vi "Det_Lock_Unlock.vi"(8 "entrée d'erreur (pas d'erreur)":errorcluster, 10 "Control-Client old entrée":refnum<class "Control-Client.lvclass">, 11 "Control-Client new entrée":refnum<class "Control-Client.lvclass">) -> (0 "sortie d'erreur":errorcluster, 2 "Control-Client old out":refnum<class "Control-Client.lvclass">, 3 "Control-Client new out":refnum<class "Control-Client.lvclass">)   [LabVIEW 2019, in "Control-Client.lvclass"]
uses:
  Control-Client.lvclass
  Control-Client.lvclass/Control-Client.ctl
  controls/Gauge_pump/Gauge_pump.xctl
  dependecies/XControls/CellsDL/ControlDL.xctl
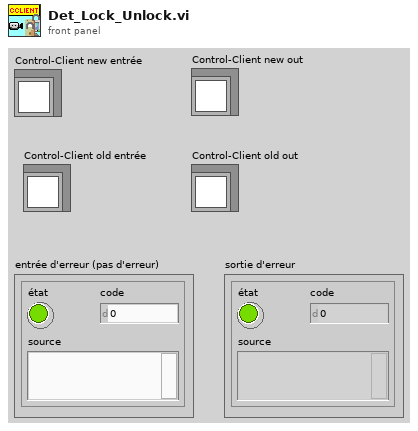
[diagram p1: front panel]
types:
  T1 = enum8{"Enabled", "Disabled", "Disabled and Grayed Out"}
  T2 = typedef "Control-Client.lvclass/Controls-with-permissions_CLIENT.ctl" = cluster{"Server ON/OFF":refnum<vi>, "Detector connect":refnum<vi>, "DL connect":refnum<vi>, "DAQmx connect":refnum<vi>, "All connect":refnum<vi>, "Start measurement":refnum<vi>, "Move Crystal":refnum<vi>, "Relay key heater":refnum<vi>, "Laser Shutter":refnum<vi>, "Accelerator Shutter":refnum<vi>, "Power":refnum<vi>, "Unlock":refnum<vi>, "RT":refnum<vi>, "Faraday Cup":refnum<vi>, "Osc connect":refnum<vi>, "ELYSE pulses":refnum<vi>, "Cells":refnum<vi>, "Pump":refnum<vi>, "# par point":refnum<vi>, "Alarm":refnum<vi>, "oscilloscopeRead":refnum<vi>, "WCM_state":refnum<vi>, "ControlDL":refnum<vi>}
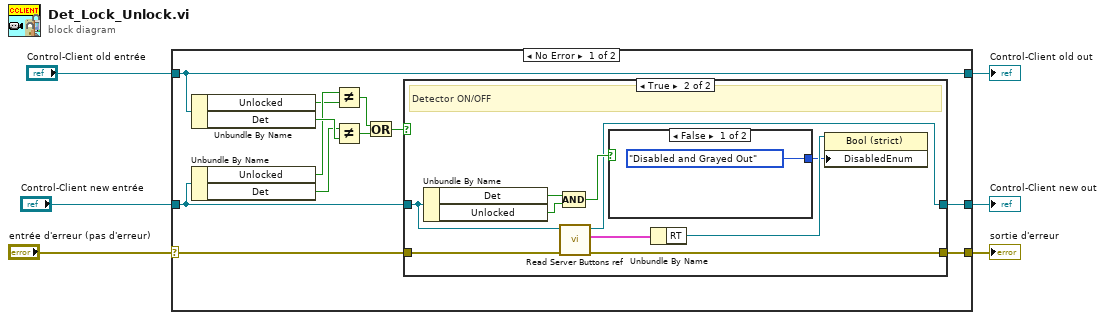
[diagram p0: block diagram]
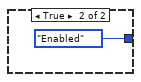
[diagram p3: hidden frame]
diagram:
  n1 = case shown="No Error" "entrée d'erreur (pas d'erreur)" {
    selector: "entrée d'erreur (pas d'erreur)" -> [w8 w33]
    tunnel: [w18 w33] -> w6
    tunnel: "Control-Client new entrée" -> [w17 w35]
    tunnel: "Control-Client old entrée" -> [w7 w34]
    tunnel: [w9 w35] -> w3
    tunnel: [w7 w34] -> w1
    frame No Error {
      n2 = Unbundle By Name(w7) -> ("Unlocked"=w10:bool, "Det"=w16:bool)
      n3 = Unbundle By Name(w17) -> ("Unlocked"=w11:bool, "Det"=w15:bool)
      n4 = Not Equal?(x=w11, y=w10) -> (x != y?=w14:bool)
      n5 = Not Equal?(x=w15, y=w16) -> (x != y?=w13:bool)
      n6 = Or(x=w14, y=w13) -> (x .or. y?=w12:bool)
      n7 = case shown="True" w12 {
        tunnel: w17 -> [w19 w24]
        tunnel: [w20 w27] -> w18
        tunnel: w8 -> [w20 w26]
        tunnel: [w19 w21] -> w9
        frame False {
        }
        frame True {
          # "Detector ON/OFF"
          n8 = Unbundle By Name(w24) -> ("Det"=w23:bool, "Unlocked"=w22:bool)
          n9 = call "Read Server Buttons ref.vi"("error in (no error)"=w26, "Control-Client in"=w24) -> ("error out"=w27:errorcluster, "Server Buttons ref"=w29:T2, "Control-Client out"=w21:refnum<class "Control-Client.lvclass">)  [unwired: 7 in]
          n10 = Compound Arithmetic op=AND(w23, w22) -> (w25:bool)
          n11 = case shown="False" w25 {
            tunnel: [T1."Disabled and Grayed Out" ("Désactivé") T1."Enabled" ("Désactivé")] -> w28
            frame False {
            }
            frame True {
            }
          }
          n12 = Unbundle By Name(w29) -> ("RT"=w30:refnum<vi>)
          n13 = property class="Bool (strict)"(reference=w30, "DisabledEnum"=w28) -> ()  [unwired: 1 in, 2 out]
        }
      }
    }
    frame Error {
    }
  }
  "sortie d'erreur" <- w6
  "Control-Client new out" <- w3
  "Control-Client old out" <- w1
